vi "ma_timeStamp.vi"(4 "dt":dbl format="%0.2f", 6 "t0":timestamp format="%<%I:%M:%S%4u %p>T", 7 "reset":bool, 9 "Number of blocks":i32, 11 "state info":T1 {"buffer" format="%0.2f"; "timestamp" format="%<%.4X>T"; "dt history" format="%0.2f"; "t0 history" format="%<%I:%M:%S%4u %p>T"; "exp TC (samples)" format="%0.2f"; "RMS history" format="%0.2f"; "DC history" format="%0.2f"}) -> (1 "dt":dbl format="%0.2f", 2 "t0":timestamp format="%<%I:%M:%S%4u %p>T", 3 "state info":T1 {"buffer" format="%0.2f"; "timestamp" format="%<%.4X>T"; "dt history" format="%0.2f"; "t0 history" format="%<%I:%M:%S%4u %p>T"; "exp TC (samples)" format="%0.2f"; "RMS history" format="%0.2f"; "DC history" format="%0.2f"})   [LabVIEW 2020, in "NI_MAPro.lvlib"]
uses:
  NI_MAPro.lvlib
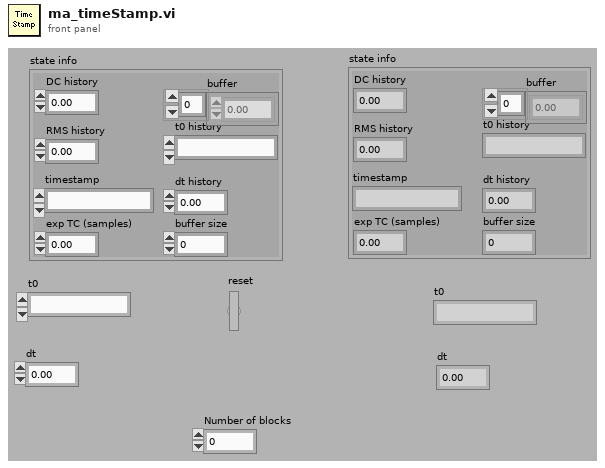
[diagram p1: front panel]
types:
  T1 = cluster{"DC history":dbl, "RMS history":dbl, "exp TC (samples)":dbl, "buffer size":i32, "t0 history":timestamp, "dt history":dbl, "timestamp":timestamp, "buffer":dbl[]}
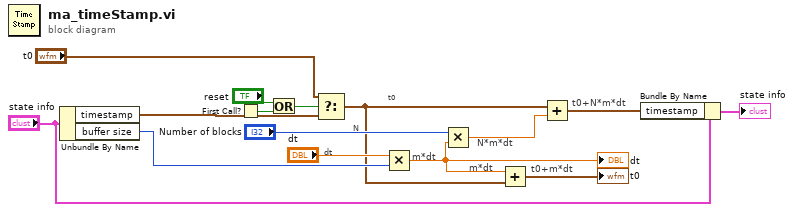
[diagram p0: block diagram]
diagram:
  # "t0+m*dt"
  # "m*dt"
  # "t0+N*m*dt"
  # "t0"
  # "N*m*dt"
  # "N"
  # "m*dt"
  # "dt"
  n1 = Unbundle By Name("state info") -> ("timestamp"=w7:timestamp, "buffer size"=w6:i32)
  n2 = First Call?() -> (First Call?: T/F=w14:bool)
  n3 = Or(x="reset", y=w14) -> (x .or. y?=w13:bool)
  n4 = Select(t="t0", s=w13, f=w7) -> (s? t:f=w2:timestamp)
  n5 = Multiply(x="dt", y=w6) -> (x*y=w1:dbl)
  "dt" <- w1
  n6 = Multiply(x="Number of blocks", y=w1) -> (x*y=w8:dbl)
  n7 = Add(x=w1, y=w2) -> (x+y=→"t0":timestamp)
  n8 = Add(x=w2, y=w8) -> (x+y=w4:timestamp)
  n9 = Bundle By Name(cluster="state info", "timestamp"=w4) -> (→"state info":T1)
